vi "rad_Format Application Images Information.vi"(11 "App Images Information":T1[](array[typedef])) -> (3 "App Images Information":string[][](array[string]))   [LabVIEW 2014]
uses:
  rad_Globals.vi
  TypeDefs/rad_Application Image Properties.ctl
  TypeDefs/rad_AppImage Information.ctl
  TypeDefs/rad_FPGA Properties.ctl
  TypeDefs/rad_FPGA Flash Properties.ctl
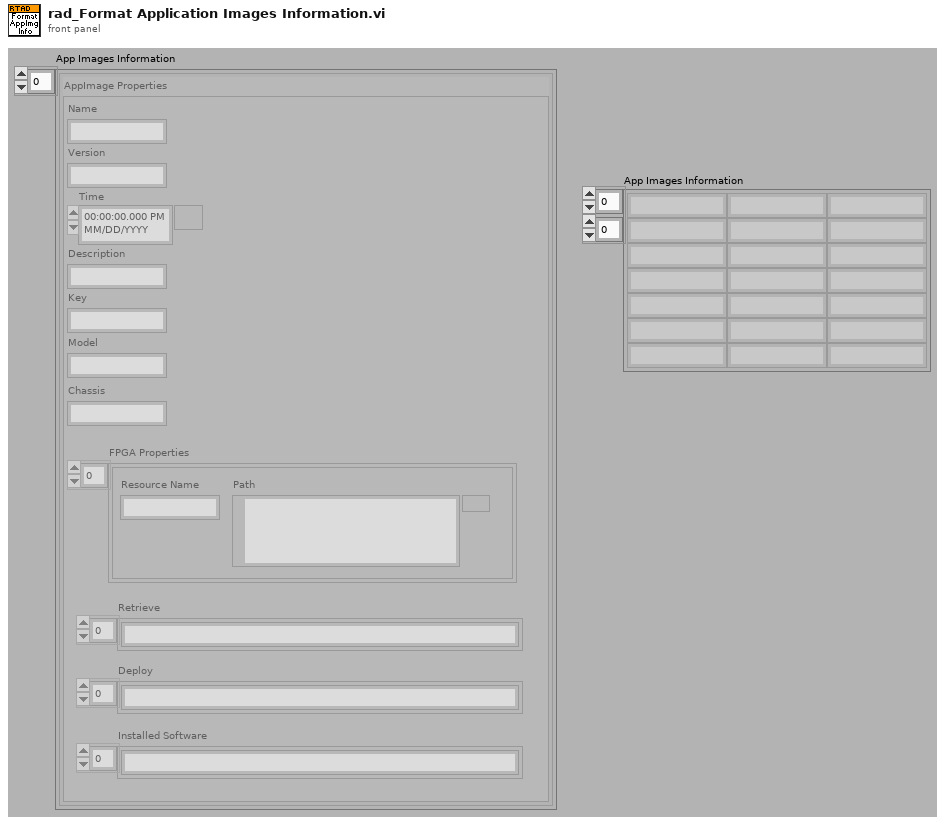
[diagram p1: front panel]
types:
  T1 = typedef "rad_AppImage Information.ctl" = cluster{"AppImage Properties":T2, "AppImage Path":path}
  T2 = typedef "rad_Application Image Properties.ctl" = cluster{"Name":string, "Version":string, "Time":timestamp, "Description":string, "Key":string, "Chassis":string, "FPGA Properties":T3, "Model":string, "Retrieve":string[], "Deploy":string[], "Installed Software":string[]}
  T3 = typedef "rad_FPGA Properties.ctl" = T4[]
  T4 = typedef "rad_FPGA Flash Properties.ctl" = cluster{"Resource Name":string, "Path":path}
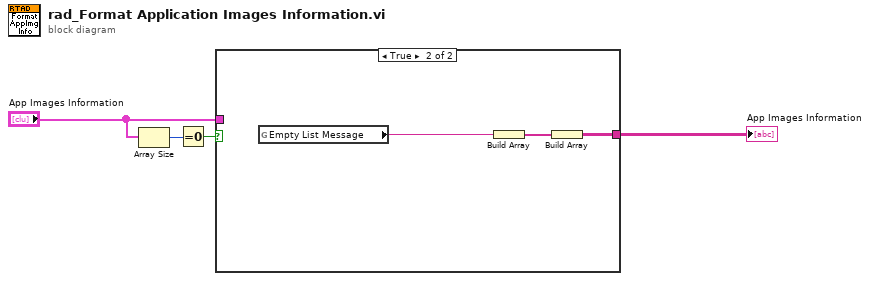
[diagram p0: block diagram]
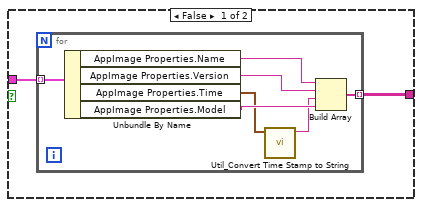
[diagram p2: hidden frame]
diagram:
  n1 = Array Size(array="App Images Information") -> (size(s)=w2:i32)
  n2 = Equal To 0?(x=w2) -> (x = 0?=w1:bool)
  n3 = case shown="True" w1 {
    tunnel: [w6 w15] -> w4
    tunnel: "App Images Information" -> [w5 _]
    frame False {
      n4 = for {
        tunnel: w5 -> [w13] mode=indexing
        tunnel: [w9] -> w6 mode=indexing
        n5 = Unbundle By Name(w13) -> ("AppImage Properties.Name"=w12:string, "AppImage Properties.Version"=w11:string, "AppImage Properties.Time"=w8:timestamp, "AppImage Properties.Model"=w10:string)
        n6 = call "Util_Convert Time Stamp to String.vi"("Time"=w8) -> ("Time"=w7:string)  [unwired: 10 out]
        n7 = Build Array(w12, w11, w7, w10) -> (w9:string[])
      }
    }
    frame True {
      n8 = global read "rad_Globals.vi" "Empty List Message"() -> (w14:string)
      n9 = Build Array(w14) -> (w16:string[])
      n10 = Build Array(w16) -> (w15:string[][])
    }
  }
  "App Images Information" <- w4
